vi "Get Focus Parameter Info.vi"(8 "error in (no error)":errorcluster, 11 "Stream in":refnum<class "Stream.lvclass">) -> (0 "error out":errorcluster, 2 "Info":T1, 3 "Stream (Duplicate)":refnum<class "Stream.lvclass">)   [LabVIEW 2020, in "g_ar_toolkit.capture.lvlib" / "Stream.lvclass"]
uses:
  Stream.lvclass
  Camera Parameter Information.ctl
  Camera Parameters.ctl
  Stream.lvclass/Stream.ctl
  g_ar_toolkit.common/Module Path.vi
  <vilib>/Utility/error.llb/Error Cluster From Error Code.vi
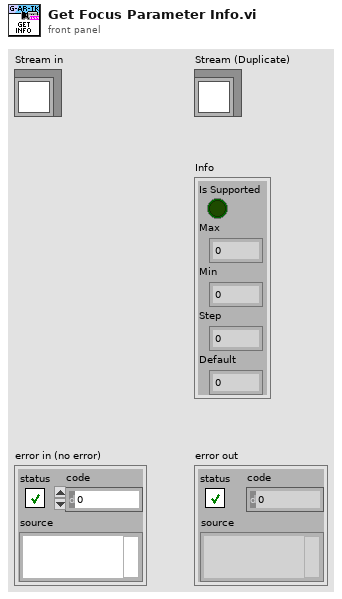
[diagram p1: front panel]
types:
  T1 = typedef "g_ar_toolkit.capture.lvlib/Stream.lvclass/Camera Parameter Information.ctl" = cluster{"Is Supported":bool, "Max":i32, "Min":i32, "Step":i32, "Default":i32}
  T2 = typedef "g_ar_toolkit.capture.lvlib/Stream.lvclass/Camera Parameters.ctl" = enum8{"EXPOSURE", "FOCUS", "ZOOM", "GAIN", "WHITE_BALANCE_TEMPERATURE", "BRIGHTNESS", "CONTRAST", "SATURATION", "GAMMA", "HUE", "SHARPNESS", "BACKLIGHT_COMPENSATION", "POWER_LINE_FREQUENCY"}
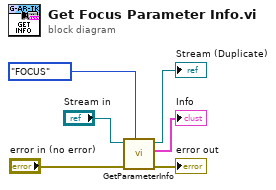
[diagram p0: block diagram]
diagram:
  n1 = call "GetParameterInfo.vi"("Camera Parameter"=Camera_Parameters."FOCUS", "error in (no error)"="error in (no error)", "Stream in"="Stream in") -> ("error out"=→"error out":errorcluster, "Info"=→"Info":T1, "Stream (Duplicate)"=→"Stream (Duplicate)":refnum<class "Stream.lvclass">)  [unwired: 6 in]
